vi "ex_6_odczyt_z_pliku_v2.vi"() -> ()   [LabVIEW 2020]
uses:
  #typedef_ProgramData.ctl
  #typedef_Product.ctl
panel:
  out "output cluster":T1
  in  "Path":path
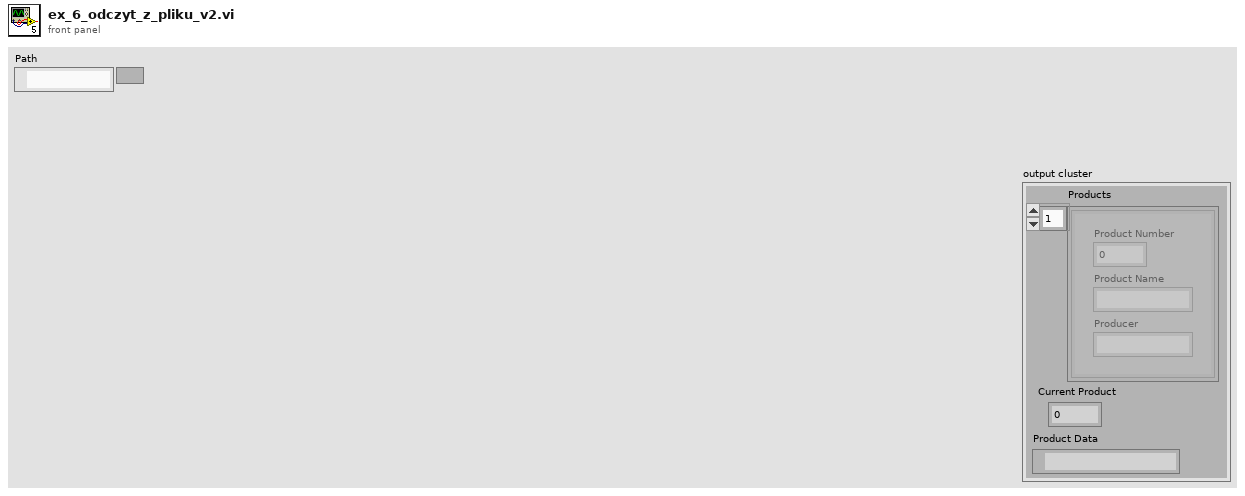
[diagram p1: front panel]
types:
  T1 = typedef "#typedef_ProgramData.ctl" = cluster{"Products":T2[], "Current Product":i32, "Product Data":path}
  T2 = typedef "#typedef_Product.ctl" = cluster{"Product Number":i32, "Product Name":string, "Producer":string}
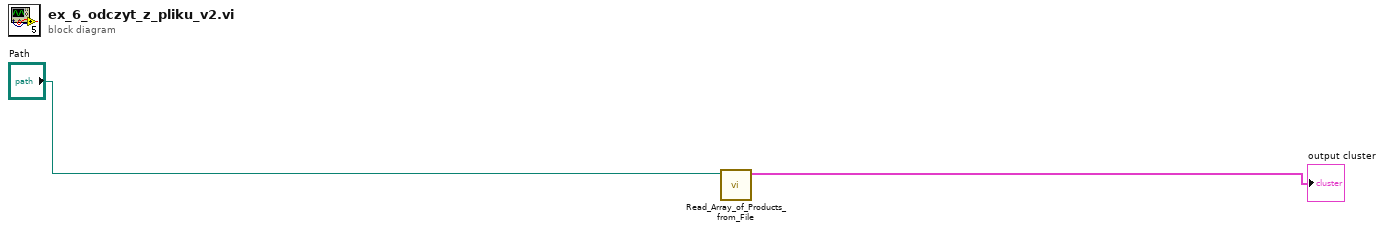
[diagram p0: block diagram]
diagram:
  n1 = call "Read_Array_of_Products_from_File.vi"("Path"="Path") -> ("Program Data"=→"output cluster":T1)  [unwired: 10 in]
